vi "Calc Force vector.vi"(2 "Pdyn ref (Pa)":sgl, 3 "Cp distribution (time averaged)":cluster{"x/c flap (sorted)":sgl[], sgl[]}[](graph)) -> (0 "Fy (N)":sgl, 1 "Fx (N)":sgl)   [LabVIEW 2015]
panel:
  in  "Area vectors, flap (sorted)":sgl[][](array[numeric])=[[-0.030221105, 0.0050799865], [-0.025013696, 0.010133014], [-0.016425999, 0.015131993], [-0.004751401, 0.020000994], [0.0092555005, 0.009600005], [0.011616802, -0.009600005], [0.017089, -0.020627992], [0.038450897, -0.029717995]]
  in  "Area vectors, wing (sorted)":sgl[][](array[numeric])=[[-0.0203481, 0.080010995], [-0.0011855003, 0.03999], [0.0039664, 0.039116003], [0.0067474004, 0.030846998], [0.007422101, 0.019963002], [0.005573, 0.009961], [0.0017389987, 0.0023479997], [0.0026417004, 0.0030260002], [0.0037459005, 0.003527], [0.0068250997, 0.002781997], [0.0076412004, -0.0055579967], [0.0006181995, -0.0030020003], [-1.3899662e-05, -0.0030160001], [-0.0003820001, -0.0030109999], [-0.0011917998, -0.006011999], [-0.0017578002, -0.0068530007], [-0.0058059003, -0.022149], [-0.0077515002, -0.039984], [-0.0046135993, -0.039992005], [-0.0017817, -0.03999], [0.0030151003, -0.03999099], [-0.0051033013, -0.022013]]
  # "Paste in values from geometry prep vi and make default. Delete z column."
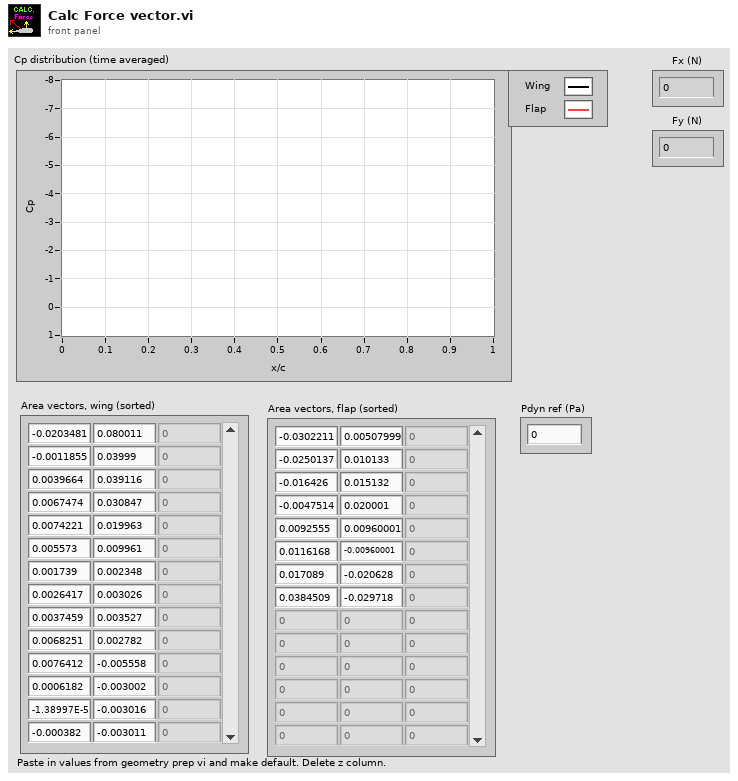
[diagram p1: front panel]
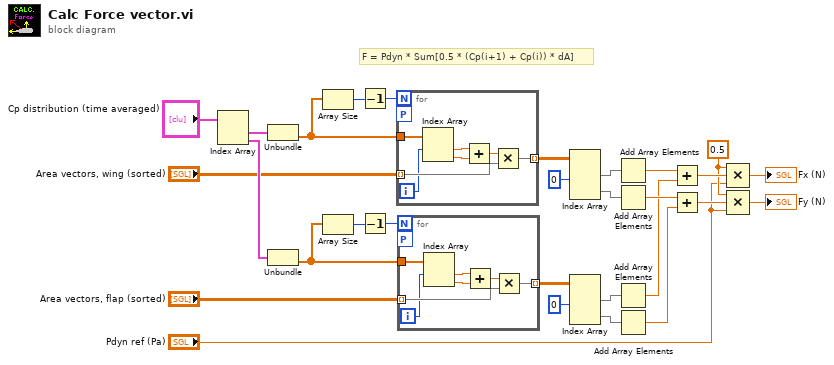
[diagram p0: block diagram]
diagram:
  w3 = sgl 0.5 ("y")
  # "F = Pdyn * Sum[0.5 * (Cp(i+1) + Cp(i)) * dA]"
  n1 = Index Array(array="Cp distribution (time averaged)") -> (element #1=w28:cluster{"x/c flap (sorted)":sgl[], sgl[]}, element #2=w27:cluster{"x/c flap (sorted)":sgl[], sgl[]})  [unwired: 2 in]
  n2 = Unbundle(w28) -> (w24:sgl[])  [unwired: 1 out]
  n3 = Unbundle(w27) -> (w20:sgl[])  [unwired: 1 out]
  n4 = Array Size(array=w24) -> (size(s)=w26:i32)
  n5 = Array Size(array=w20) -> (size(s)=w22:i32)
  n6 = Decrement(x=w26) -> (x-1=w25:i32)
  n7 = Decrement(x=w22) -> (x-1=w21:i32)
  n8 = for {
    N: w25 -> [_]
    tunnel: w24 -> [w36]
    tunnel: "Area vectors, wing (sorted)" -> [w31] mode=indexing
    workers-P: _ -> [_]
    tunnel: [w33] -> w23 mode=indexing
    i -> [w30]
    n9 = Index Array(array=w36, index #1=w30) -> (element #1=w35:sgl, element #2=w34:sgl)  [unwired: 1 in]
    n10 = Add(x=w35, y=w34) -> (x+y=w32:sgl)
    n11 = Multiply(x=w32, y=w31) -> (x*y=w33:sgl[])
  }
  n12 = for {
    N: w21 -> [_]
    tunnel: w20 -> [w43]
    tunnel: "Area vectors, flap (sorted)" -> [w38] mode=indexing
    workers-P: _ -> [_]
    tunnel: [w40] -> w11 mode=indexing
    i -> [w37]
    n13 = Index Array(array=w43, index #1=w37) -> (element #1=w42:sgl, element #2=w41:sgl)  [unwired: 1 in]
    n14 = Add(x=w42, y=w41) -> (x+y=w39:sgl)
    n15 = Multiply(x=w39, y=w38) -> (x*y=w40:sgl[])
  }
  n16 = Index Array(array=w23, index (col) #1=0 ("disabled index (col)")) -> (element #1=w16:sgl[], element #2=w15:sgl[])  [unwired: 3 in]
  n17 = Index Array(array=w11, index (col) #1=0 ("disabled index (col)")) -> (element #1=w13:sgl[], element #2=w14:sgl[])  [unwired: 3 in]
  n18 = Add Array Elements(numeric array=w16) -> (sum=w7:sgl)
  n19 = Add Array Elements(numeric array=w15) -> (sum=w10:sgl)
  n20 = Add Array Elements(numeric array=w13) -> (sum=w8:sgl)
  n21 = Add Array Elements(numeric array=w14) -> (sum=w9:sgl)
  n22 = Add(x=w7, y=w8) -> (x+y=w6:sgl)
  n23 = Add(x=w10, y=w9) -> (x+y=w4:sgl)
  n24 = Compound Arithmetic op=MULTIPLY(w3, w6, "Pdyn ref (Pa)") -> (→"Fx (N)":sgl)
  n25 = Compound Arithmetic op=MULTIPLY(w3, w4, "Pdyn ref (Pa)") -> (→"Fy (N)":sgl)
